vi "ExTestPutRowU16.vi"() -> ()   [LabVIEW 2010]
panel:
  out "Image Display 2":u16[][](graph)
  out "error out":errorcluster
  in  "error in (no error)":errorcluster
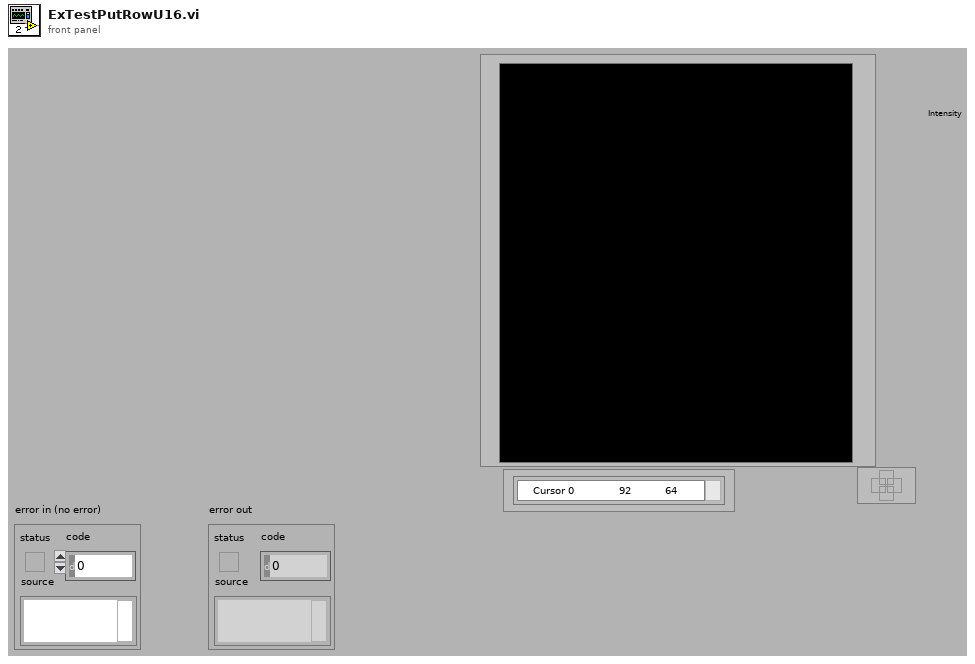
[diagram p1: front panel]
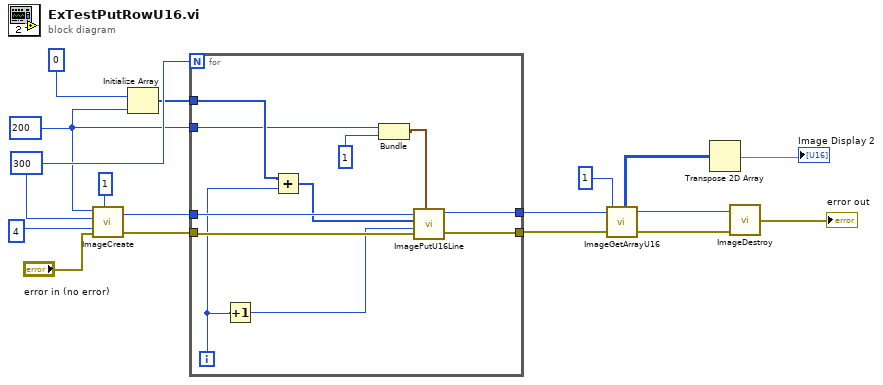
[diagram p0: block diagram]
diagram:
  w4 = 200
  w15 = 300
  n1 = call <userlib>:"ImageCreate.vi"("X dimension"=w4, "Y dimension"=w15, "Data Type"=4, "error in"="error in (no error)", "Number Of Frames"=1) -> ("Image Handle"=w5:u32, "error out"=w7:errorcluster)
  n2 = Initialize Array(u16 0, w4) -> (w6:u16[])
  n3 = for {
    N: w15 -> [_]
    tunnel: w7 -> [w28]
    tunnel: w6 -> [w26]
    tunnel: w5 -> [w22]
    tunnel: w4 -> [w25]
    tunnel: [w23] -> w2
    tunnel: [w18] -> w1
    i -> [w21]
    n4 = Increment(x=w21) -> (x+1=w27:i32)
    n5 = Add(x=w26, y=w21) -> (x+y=w20:i32[])
    n6 = Bundle(w25, 1) -> (w19:cluster{i32, i32})  [unwired: 1 in]
    n7 = call <userlib>:"ImagePutU16Line.vi"("Image Handle"=w22, "Image Data"=w20, "Y Position"=w27, "error in (no error)"=w28, "Image dimensions"=w19) -> ("Image Handle"=w23:u32, "error out"=w18:errorcluster)
  }
  n8 = call <userlib>:"ImageGetArrayU16.vi"("error in"=w1, "Z position"=1, "Image Handle"=w2) -> ("error out"=w3:errorcluster, "Array uint 16"=w11:u16[][], "Image Handle"=w9:u32)
  n9 = Transpose 2D Array(2D array=w11) -> (transposed array=→"Image Display 2":u16[][])
  n10 = call <userlib>:"ImageDestroy.vi"("error in"=w3, "Data handle"=w9) -> ("error out"=→"error out":errorcluster)
